vi "UI_Set_Play_State_(03A).vi"(3 "error in (no error)":errorcluster, 4 "Settings cluster in":T1={"Defaults"={"Default User"=0.0, "VISA Resource Name "=""}, "Recording and saving"={"Researcher name"="", "Name prefix"="", "Data filtering"=0, "Stop at"=0.0, "\"Stop at\" enabled"=FALSE}, "Geometry"={"Cage diameter, mm"=0, "Starting angle MIDFIELD"=0, "Starting angle BORDER"=0, "Radius, mm CENTER"=0, "Radius, mm MIDFIELD"=0, "N segments MIDFIELD"=0, "N segments BORDER"=0, "R-gap, mm"=0.0, "Bridge swap"=FALSE, "Bridge H. offset"=0.0, "Bridge V. offset"=0.0, "Twisted neck"=FALSE, "Alt. magn. orientation"=FALSE}, "IO parameters"={"IO general config."=0, "IO 1 configuration"=0, "IO 2 configuration"=0, "IO 3 configuration"=0, "IO 4 configuration"=0, "Activate ext. RS-232"=0, "IO inversion config."=0, "Sync capability"=1}, "Stimulus presets array"=[{"Event type"=0, "Dur., s"=0.0, "Stim., s"=0.0, "TTL out N"=1, "Set/Clear"=FALSE, "Stim. has been set"=FALSE}, {"Event type"=0, "Dur., s"=0.0, "Stim., s"=0.0, "TTL out N"=1, "Set/Clear"=FALSE, "Stim. has been set"=FALSE}, {"Event type"=0, "Dur., s"=0.0, "Stim., s"=0.0, "TTL out N"=1, "Set/Clear"=FALSE, "Stim. has been set"=FALSE}, {"Event type"=0, "Dur., s"=0.0, "Stim., s"=0.0, "TTL out N"=1, "Set/Clear"=FALSE, "Stim. has been set"=FALSE}, {"Event type"=0, "Dur., s"=0.0, "Stim., s"=0.0, "TTL out N"=1, "Set/Clear"=FALSE, "Stim. has been set"=FALSE}, {"Event type"=0, "Dur., s"=0.0, "Stim., s"=0.0, "TTL out N"=1, "Set/Clear"=FALSE, "Stim. has been set"=FALSE}, {"Event type"=0, "Dur., s"=0.0, "Stim., s"=0.0, "TTL out N"=1, "Set/Clear"=FALSE, "Stim. has been set"=FALSE}, {"Event type"=0, "Dur., s"=0.0, "Stim., s"=0.0, "TTL out N"=1, "Set/Clear"=FALSE, "Stim. has been set"=FALSE}, {"Event type"=0, "Dur., s"=0.0, "Stim., s"=0.0, "TTL out N"=1, "Set/Clear"=FALSE, "Stim. has been set"=FALSE}, {"Event type"=0, "Dur., s"=0.0, "Stim., s"=0.0, "TTL out N"=1, "Set/Clear"=FALSE, "Stim. has been set"=FALSE}, {"Event type"=0, "Dur., s"=0.0, "Stim., s"=0.0, "TTL out N"=1, "Set/Clear"=FALSE, "Stim. has been set"=FALSE}, {"Event type"=0, "Dur., s"=0.0, "Stim., s"=0.0, "TTL out N"=1, "Set/Clear"=FALSE, "Stim. has been set"=FALSE}, {"Event type"=0, "Dur., s"=0.0, "Stim., s"=0.0, "TTL out N"=1, "Set/Clear"=FALSE, "Stim. has been set"=FALSE}, {"Event type"=0, "Dur., s"=0.0, "Stim., s"=0.0, "TTL out N"=1, "Set/Clear"=FALSE, "Stim. has been set"=FALSE}], "Settings loaded OK"=FALSE} {"Stimulus presets array"."Event type" items=["Stay for N seconds"]; "Stimulus presets array"."TTL out N" items=["1"=1, "2"=2, "1+2"=3]; "Geometry"."Cage diameter, mm" scale=0.0..340.0}, 5 "All references in":T7) -> (0 "error out":errorcluster, 1 "Settings cluster out":T1={"Defaults"={"Default User"=0.0, "VISA Resource Name "=""}, "Recording and saving"={"Researcher name"="", "Name prefix"="", "Data filtering"=0, "Stop at"=0.0, "\"Stop at\" enabled"=FALSE}, "Geometry"={"Cage diameter, mm"=0, "Starting angle MIDFIELD"=0, "Starting angle BORDER"=0, "Radius, mm CENTER"=0, "Radius, mm MIDFIELD"=0, "N segments MIDFIELD"=0, "N segments BORDER"=0, "R-gap, mm"=0.0, "Bridge swap"=FALSE, "Bridge H. offset"=0.0, "Bridge V. offset"=0.0, "Twisted neck"=FALSE, "Alt. magn. orientation"=FALSE}, "IO parameters"={"IO general config."=0, "IO 1 configuration"=0, "IO 2 configuration"=0, "IO 3 configuration"=0, "IO 4 configuration"=0, "Activate ext. RS-232"=0, "IO inversion config."=0, "Sync capability"=1}, "Stimulus presets array"=[{"Event type"=0, "Dur., s"=0.0, "Stim., s"=0.0, "TTL out N"=1, "Set/Clear"=FALSE, "Stim. has been set"=FALSE}, {"Event type"=0, "Dur., s"=0.0, "Stim., s"=0.0, "TTL out N"=1, "Set/Clear"=FALSE, "Stim. has been set"=FALSE}, {"Event type"=0, "Dur., s"=0.0, "Stim., s"=0.0, "TTL out N"=1, "Set/Clear"=FALSE, "Stim. has been set"=FALSE}, {"Event type"=0, "Dur., s"=0.0, "Stim., s"=0.0, "TTL out N"=1, "Set/Clear"=FALSE, "Stim. has been set"=FALSE}, {"Event type"=0, "Dur., s"=0.0, "Stim., s"=0.0, "TTL out N"=1, "Set/Clear"=FALSE, "Stim. has been set"=FALSE}, {"Event type"=0, "Dur., s"=0.0, "Stim., s"=0.0, "TTL out N"=1, "Set/Clear"=FALSE, "Stim. has been set"=FALSE}, {"Event type"=0, "Dur., s"=0.0, "Stim., s"=0.0, "TTL out N"=1, "Set/Clear"=FALSE, "Stim. has been set"=FALSE}, {"Event type"=0, "Dur., s"=0.0, "Stim., s"=0.0, "TTL out N"=1, "Set/Clear"=FALSE, "Stim. has been set"=FALSE}, {"Event type"=0, "Dur., s"=0.0, "Stim., s"=0.0, "TTL out N"=1, "Set/Clear"=FALSE, "Stim. has been set"=FALSE}, {"Event type"=0, "Dur., s"=0.0, "Stim., s"=0.0, "TTL out N"=1, "Set/Clear"=FALSE, "Stim. has been set"=FALSE}, {"Event type"=0, "Dur., s"=0.0, "Stim., s"=0.0, "TTL out N"=1, "Set/Clear"=FALSE, "Stim. has been set"=FALSE}, {"Event type"=0, "Dur., s"=0.0, "Stim., s"=0.0, "TTL out N"=1, "Set/Clear"=FALSE, "Stim. has been set"=FALSE}, {"Event type"=0, "Dur., s"=0.0, "Stim., s"=0.0, "TTL out N"=1, "Set/Clear"=FALSE, "Stim. has been set"=FALSE}, {"Event type"=0, "Dur., s"=0.0, "Stim., s"=0.0, "TTL out N"=1, "Set/Clear"=FALSE, "Stim. has been set"=FALSE}], "Settings loaded OK"=FALSE} {"Stimulus presets array"."Event type" items=["Stay for N seconds"]; "Stimulus presets array"."TTL out N" items=["1"=1, "2"=2, "1+2"=3]; "Geometry"."Cage diameter, mm" scale=0.0..340.0}, 2 "All references out":T7)   [LabVIEW 2018]
uses:
  Controls/CTL_All_References.ctl
  Controls/CTL_Controls_References.ctl
  Controls/CTL_Indicators_References.ctl
  Controls/CTL_Panes_and_VIs_References.ctl
  Controls/CTL_Histogram_Properties.ctl
  <vilib>/Utility/miscctls.llb/LVRangeTypeDef.ctl
  Controls/CTL_Settings_cluster.ctl
  Controls/CTL_Segmented_plot_parameters.ctl
  Controls/CTL_IO_params_cluster.ctl
  Controls/CTL_Single_stimulus_setting.ctl
  <vilib>/Utility/error.llb/Error Cluster From Error Code.vi
  <vilib>/ErrorRing/Error Ring.xnode
panel:
  in  "Histogram initialization cluster":T5={"X Scale.Range"={"Minimum"=0.0, "Maximum"=13.0, "Increment"=1.0, "Minor Increment"=1.0, "Start"=0.0}, "Caption.Text"="Zone preference (normalized)", "X Scale.Offset and Multiplier:Multiplier"=1.0, "X Scale.Offset and Multiplier:Offset"=0.0, "X Scale.Scale Fit"=2, "X Scale.Display Format:Precision"=0, "Y Scale.Mapping Mode"=0, "Zones preference empty initialized array"=[0, 0, 0, 0, 0, 0, 0, 0, 0, 0, 0, 0, 0, 0], "Plot.Fill/Point Color"=15790320}
  out "Panes references":T10
  out "Controls references params":string[][](array[string])
  out "Indicators references params":string[][](array[string])
  out "Indicators references":T9
  out "Controls references":T8
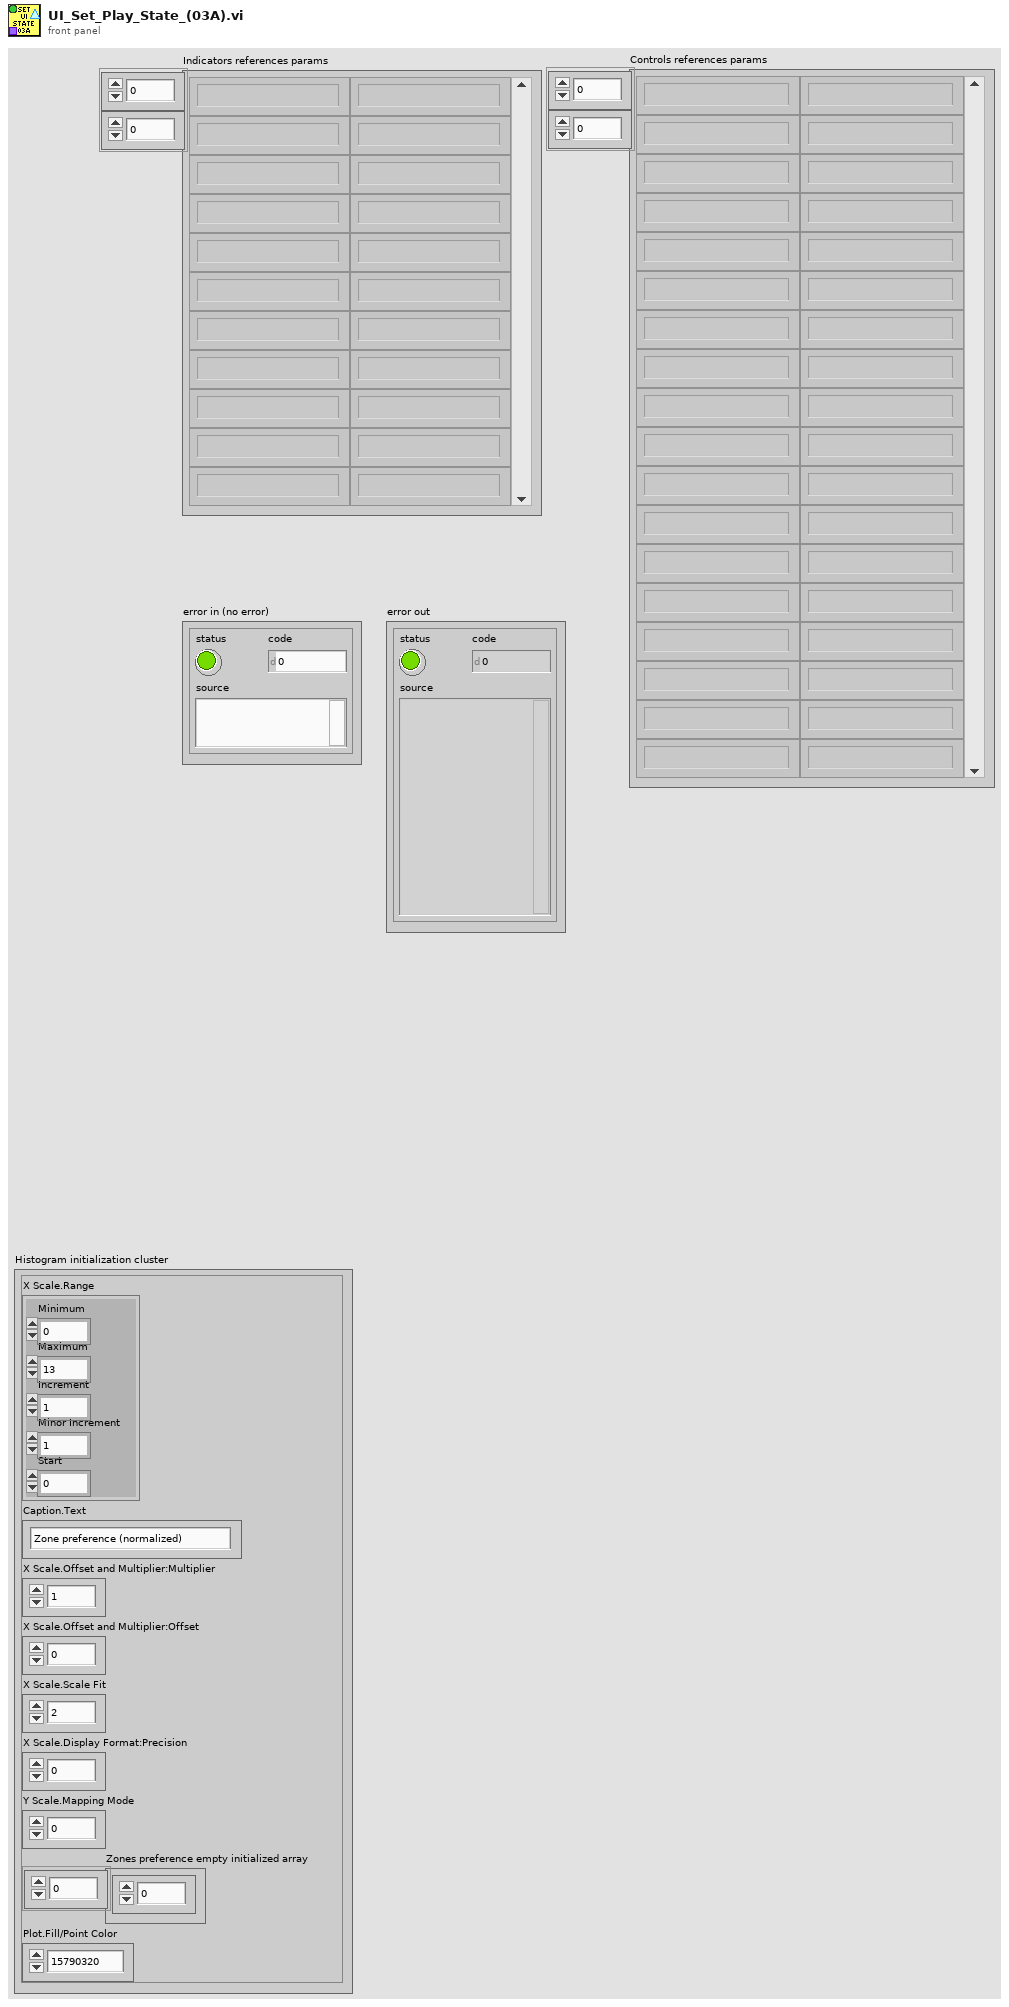
[diagram p1: front panel]
types:
  T1 = typedef "CTL_Settings_cluster.ctl" = cluster{"Defaults":cluster{"Default User":dbl, "VISA Resource Name ":string}, "Recording and saving":cluster{"Researcher name":string, "Name prefix":string, "Data filtering":u16, "Stop at":dbl, "\"Stop at\" enabled":bool}, "Geometry":T2, "IO parameters":T3, "Stimulus presets array":T4[], "Settings loaded OK":bool}
  T2 = typedef "CTL_Segmented_plot_parameters.ctl" = cluster{"Cage diameter, mm":u16, "Starting angle MIDFIELD":i16, "Starting angle BORDER":i16, "Radius, mm CENTER":u16, "Radius, mm MIDFIELD":u16, "N segments MIDFIELD":u8, "N segments BORDER":u8, "R-gap, mm":sgl, "Bridge swap":bool, "Bridge H. offset":sgl, "Bridge V. offset":sgl, "Twisted neck":bool, "Alt. magn. orientation":bool}
  T3 = typedef "CTL_IO_params_cluster.ctl" = cluster{"IO general config.":u16, "IO 1 configuration":u16, "IO 2 configuration":u16, "IO 3 configuration":u16, "IO 4 configuration":u16, "Activate ext. RS-232":u16, "IO inversion config.":u16, "Sync capability":u8}
  T4 = typedef "CTL_Single_stimulus_setting.ctl" = cluster{"Event type":u16, "Dur., s":sgl, "Stim., s":sgl, "TTL out N":u16, "Set/Clear":bool, "Stim. has been set":bool}
  T5 = typedef "CTL_Histogram_Properties.ctl" = cluster{"X Scale.Range":T6, "Caption.Text":string, "X Scale.Offset and Multiplier:Multiplier":dbl, "X Scale.Offset and Multiplier:Offset":dbl, "X Scale.Scale Fit":u8, "X Scale.Display Format:Precision":u8, "Y Scale.Mapping Mode":u8, "Zones preference empty initialized array":i32[], "Plot.Fill/Point Color":u32}
  T6 = typedef "LVRangeTypeDef.ctl" = cluster{"Minimum":dbl, "Maximum":dbl, "Increment":dbl, "Minor Increment":dbl, "Start":dbl}
  T7 = typedef "CTL_All_References.ctl" = cluster{"Controls references":T8, "Indicators references":T9, "Panes references":T10}
  T8 = typedef "CTL_Controls_References.ctl" = cluster{"Check HW connection":refnum<vi>, "Start Tracking button":refnum<vi>, "Reset zones":refnum<vi>, "Reset stimuli":refnum<vi>, "Record/Stop":refnum<vi>, "Reset barplot":refnum<vi>, "Multiplyer of chart RX":refnum<vi>, "Show zones":refnum<vi>, "Show magnets":refnum<vi>, "Show heatmap":refnum<vi>, "Show full track":refnum<vi>, "Open File":refnum<vi>, "Play/Pause":refnum<vi>, "Trace, s":refnum<vi>, "Playback speed":refnum<vi>, "Timeline":refnum<vi>, "By Zone stim. setup":refnum<vi>, "Set, Rec and Analyse Tab":refnum<vi>, "Cage radial segmentation":refnum<vi>, "Set IO config":refnum<vi>}
  T9 = typedef "CTL_Indicators_References.ctl" = cluster{"HW info":refnum<vi>, "Port":refnum<vi>, "Ready":refnum<vi>, "IO status indicator":refnum<vi>, "Current Time":refnum<vi>, "Record timestamp":refnum<vi>, "Mouse speed":refnum<vi>, "Mouse speed, mm/s":refnum<vi>, "Running, perc. of time":refnum<vi>, "Histograms":refnum<vi>, "Cage size":refnum<vi>}
  T10 = typedef "CTL_Panes_and_VIs_References.ctl" = cluster{"Pane":refnum<vi>, "This VI":refnum<vi>}
  T11 = enum8{"Enabled", "Disabled", "Disabled and Grayed Out"}
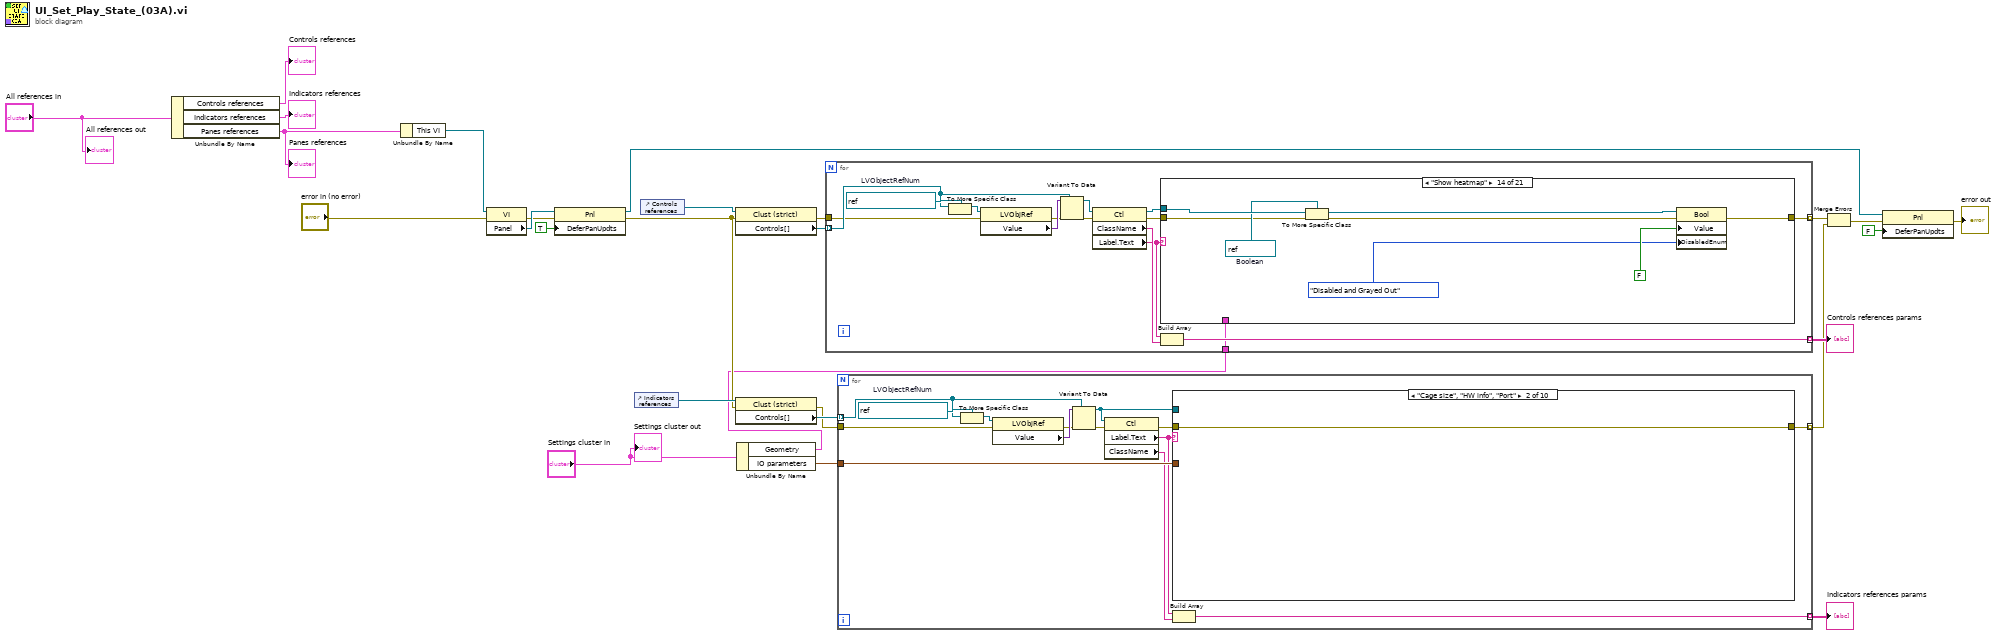
[diagram p0: block diagram]
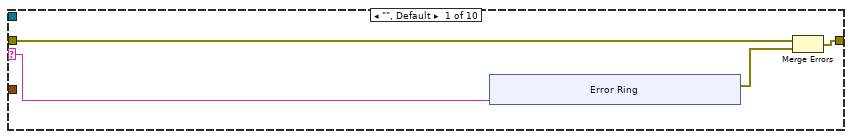
[diagram p2: hidden frame]
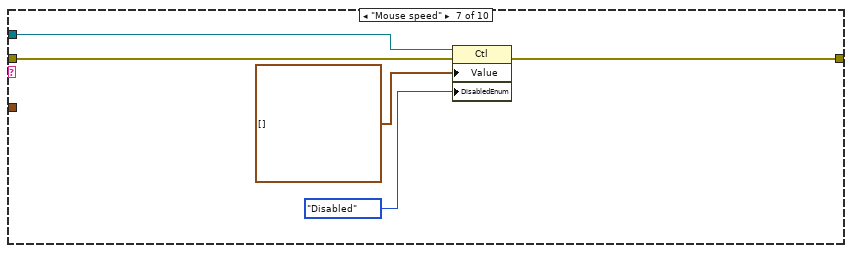
[diagram p7: hidden frame]
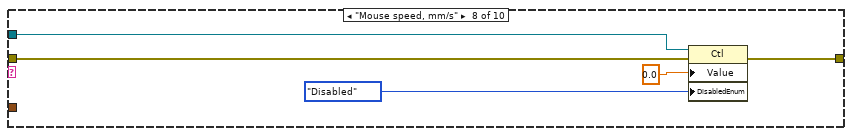
[diagram p8: hidden frame]
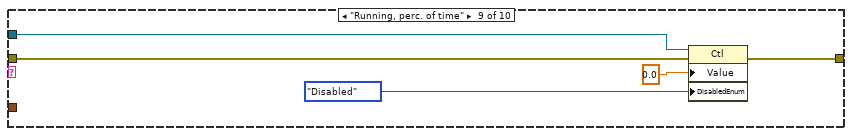
[diagram p9: hidden frame]
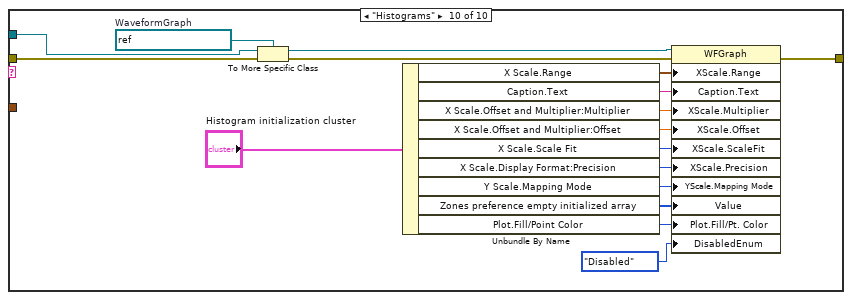
[diagram p10: hidden frame]
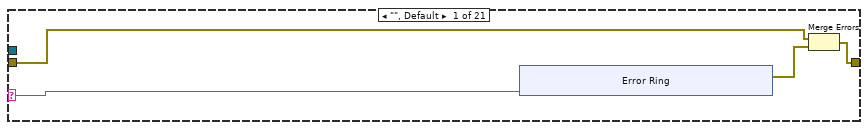
[diagram p11: hidden frame]
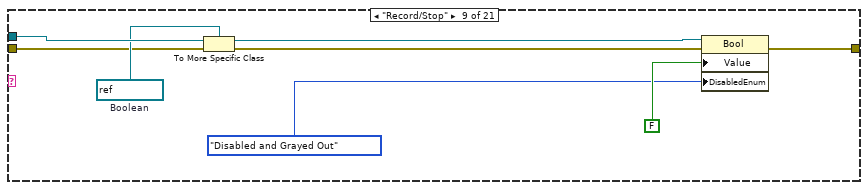
[diagram p19: hidden frame]
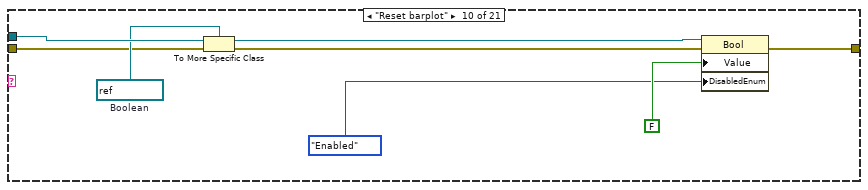
[diagram p20: hidden frame]
diagram:
  n1 = Unbundle By Name("All references in") -> ("Controls references"=→"Controls references":T8, "Indicators references"=→"Indicators references":T9, "Panes references"=w18:T10)
  "Panes references" <- w18
  n2 = Unbundle By Name(w18) -> ("This VI"=w15:refnum<vi>)
  n3 = property class="VI"(reference=w15, error in="error in (no error)") -> (error out=w7:errorcluster, "Panel"=w17:refnum<vi>)  [unwired: 1 out]
  n4 = property class="Pnl"(reference=w17, error in=w7, "DeferPanUpdts"=TRUE ("Defer Panel Updates")) -> (reference out=w8:refnum<vi>, error out=w14:errorcluster)
  n5 = control-ref of="Indicators references"() -> (w21:refnum<vi>)
  n6 = control-ref of="Controls references"() -> (w23:refnum<vi>)
  n7 = property class="Clust (strict)"(reference=w23, error in=w14) -> (error out=w13:errorcluster, "Controls[]"=w24:refnum<vi>[])  [unwired: 1 out]
  n8 = property class="Clust (strict)"(reference=w21, error in=w14) -> (error out=w12:errorcluster, "Controls[]"=w22:refnum<vi>[])  [unwired: 1 out]
  n9 = Unbundle By Name("Settings cluster in") -> ("Geometry"=w1:T2, "IO parameters"=w3:T3)
  n10 = for {
    tunnel: w24 -> [w39] mode=indexing
    tunnel: [w36] -> w19 mode=indexing
    tunnel: w13 -> [w35]
    tunnel: [w31] -> w5 mode=indexing
    tunnel: w1 -> [w28]
    w41 = refnum<vi> refnum  # LVObjectRefNum
    n11 = To More Specific Class(target class=w41, reference=w39) -> (specific class reference=w42:refnum<vi>)  [unwired: 1 in, 1 out]
    n12 = property class="LVObjRef"(reference=w42, error in=w35) -> (error out=w34:errorcluster, "Value"=w40:variant)  [unwired: 1 out]
    n13 = Variant To Data(error in=w34, type=w39, Variant=w40) -> (data=w38:refnum<vi>, error out=w33:errorcluster)
    n14 = property class="Ctl"(reference=w38, error in=w33) -> (reference out=w29:refnum<vi>, error out=w30:errorcluster, "ClassName"=w37:string, "Label.Text"=w32:string)
    n15 = case shown="\"Show heatmap\"" w32 {
      selector: w32 -> [w43 _ _ _ _ _ _ _ _ _ _ _ _ _ _ _ _ _ _ _ _]
      tunnel: [w45 w54 w55 w56 w57 w58 w59 w60 w63 w71 w79 w87 w93 w96 w104 w110 w111 w114 w122 w130 w136] -> w31
      tunnel: w30 -> [w46 w54 w55 w56 w57 w58 w59 w60 w65 w73 w81 w89 w93 w98 w106 w110 w111 w116 w124 w132 w136]
      tunnel: w29 -> [_ _ _ _ _ _ _ _ w68 w76 w84 w92 _ w101 w109 _ _ w119 w127 w135 _]
      tunnel: w28 -> [_ _ _ _ _ _ _ _ _ _ _ _ _ _ _ _ _ _ _ _ _]
      frame "", Default {
        n16 = xnode "Error Ring"("parameter 0"=w43) -> ("error out"=w44:errorcluster)
        n17 = Merge Errors(w46, w44) -> (w45:errorcluster)
      }
      frame "Cage radial segmentation" {
      }
      frame "Set/Rec and Analyse Tab" {
      }
      frame "Check HW connection" {
      }
      frame "Save settings" {
      }
      frame "Set IO config" {
      }
      frame "Reset zones" {
      }
      frame "Reset stimuli" {
      }
      frame "Record/Stop" {
        w67 = refnum<vi> refnum  # Boolean
        n18 = To More Specific Class(target class=w67, reference=w68, error in=w65) -> (specific class reference=w66:refnum<vi>, error out=w64:errorcluster)
        n19 = property class="Bool"(reference=w66, error in=w64, "Value"=FALSE, "DisabledEnum"=T11."Disabled and Grayed Out" ("Disabled")) -> (error out=w63:errorcluster)  [unwired: 1 out]
      }
      frame "Reset barplot" {
        w75 = refnum<vi> refnum  # Boolean
        n20 = To More Specific Class(target class=w75, reference=w76, error in=w73) -> (specific class reference=w74:refnum<vi>, error out=w72:errorcluster)
        n21 = property class="Bool"(reference=w74, error in=w72, "Value"=FALSE, "DisabledEnum"=T11."Enabled" ("Disabled")) -> (error out=w71:errorcluster)  [unwired: 1 out]
      }
      frame "Multiplyer of chart RX" {
        w83 = refnum<vi> refnum  # Slide
        n22 = To More Specific Class(target class=w83, reference=w84, error in=w81) -> (specific class reference=w82:refnum<vi>, error out=w80:errorcluster)
        n23 = property class="Slide"(reference=w82, error in=w80, "Value"=u8 1, "DisabledEnum"=T11."Enabled" ("Disabled")) -> (error out=w79:errorcluster)  [unwired: 1 out]
      }
      frame "Show zones" {
        w91 = refnum<vi> refnum  # Boolean
        n24 = To More Specific Class(target class=w91, reference=w92, error in=w89) -> (specific class reference=w90:refnum<vi>, error out=w88:errorcluster)
        n25 = property class="Bool"(reference=w90, error in=w88, "Value"=TRUE, "DisabledEnum"=T11."Enabled" ("Disabled")) -> (error out=w87:errorcluster)  [unwired: 1 out]
      }
      frame "Show magnets" {
      }
      frame "Show heatmap" {
        w100 = refnum<vi> refnum  # Boolean
        n26 = To More Specific Class(target class=w100, reference=w101, error in=w98) -> (specific class reference=w99:refnum<vi>, error out=w97:errorcluster)
        n27 = property class="Bool"(reference=w99, error in=w97, "Value"=FALSE, "DisabledEnum"=T11."Disabled and Grayed Out" ("Disabled")) -> (error out=w96:errorcluster)  [unwired: 1 out]
      }
      frame "Show full track" {
        w108 = refnum<vi> refnum  # Boolean
        n28 = To More Specific Class(target class=w108, reference=w109, error in=w106) -> (specific class reference=w107:refnum<vi>, error out=w105:errorcluster)
        n29 = property class="Bool"(reference=w107, error in=w105, "Value"=FALSE, "DisabledEnum"=T11."Disabled and Grayed Out" ("Disabled")) -> (error out=w104:errorcluster)  [unwired: 1 out]
      }
      frame "Open File" {
      }
      frame "Play/Pause" {
      }
      frame "Trace, s" {
        w118 = refnum<vi> refnum  # Slide
        n30 = To More Specific Class(target class=w118, reference=w119, error in=w116) -> (specific class reference=w117:refnum<vi>, error out=w115:errorcluster)
        n31 = property class="Slide"(reference=w117, error in=w115, "Value"=u8 5, "DisabledEnum"=T11."Enabled" ("Disabled")) -> (error out=w114:errorcluster)  [unwired: 1 out]
      }
      frame "Playback speed" {
        w126 = refnum<vi> refnum  # Ring
        n32 = To More Specific Class(target class=w126, reference=w127, error in=w124) -> (specific class reference=w125:refnum<vi>, error out=w123:errorcluster)
        n33 = property class="Ring"(reference=w125, error in=w123, "Value"=u8 3, "DisabledEnum"=T11."Disabled and Grayed Out" ("Disabled")) -> (error out=w122:errorcluster)  [unwired: 1 out]
      }
      frame "Timeline" {
        w134 = refnum<vi> refnum  # Slide
        n34 = To More Specific Class(target class=w134, reference=w135, error in=w132) -> (specific class reference=w133:refnum<vi>, error out=w131:errorcluster)
        n35 = property class="Slide"(reference=w133, error in=w131, "Value"=u8 5, "DisabledEnum"=T11."Disabled" ("Disabled")) -> (error out=w130:errorcluster)  [unwired: 1 out]
      }
      frame "By Zone stim. setup" {
      }
    }
    n36 = Build Array(w32, w37) -> (w36:string[])
  }
  "Controls references params" <- w19
  n37 = for {
    tunnel: w22 -> [w147] mode=indexing
    tunnel: [w137] -> w20 mode=indexing
    tunnel: w12 -> [w145]
    tunnel: [w141] -> w11 mode=indexing
    tunnel: w3 -> [w140]
    w149 = refnum<vi> refnum  # LVObjectRefNum
    n38 = To More Specific Class(target class=w149, reference=w147) -> (specific class reference=w150:refnum<vi>)  [unwired: 1 in, 1 out]
    n39 = property class="LVObjRef"(reference=w150, error in=w145) -> (error out=w144:errorcluster, "Value"=w148:variant)  [unwired: 1 out]
    n40 = Variant To Data(error in=w144, type=w147, Variant=w148) -> (data=w146:refnum<vi>, error out=w143:errorcluster)
    n41 = property class="Ctl"(reference=w146, error in=w143) -> (error out=w142:errorcluster, "Label.Text"=w139:string, "ClassName"=w138:string)  [unwired: 1 out]
    n42 = case shown="\"Cage size\", \"HW info\", \"Port\"" w139 {
      selector: w139 -> [w151 _ _ _ _ _ _ _ _ _]
      tunnel: w146 -> [_ _ _ _ _ _ w171 w176 w181 w198]
      tunnel: w142 -> [w154 w162 w163 w164 w165 w166 w170 w175 w180 w184]
      tunnel: [w153 w162 w163 w164 w165 w166 w169 w174 w179 w197] -> w141
      tunnel: w140 -> [_ _ _ _ _ _ _ _ _ _]
      frame "", Default {
        n43 = xnode "Error Ring"("parameter 0"=w151) -> ("error out"=w152:errorcluster)
        n44 = Merge Errors(w154, w152) -> (w153:errorcluster)
      }
      frame "Cage size", "HW info", "Port" {
      }
      frame "Ready" {
      }
      frame "IO status indicator" {
      }
      frame "Current Time" {
      }
      frame "Record timestamp" {
      }
      frame "Mouse speed" {
        n45 = property class="Ctl"(reference=w171, error in=w170, "Value"=waveform(dbl)[] [] ("History Data"), "DisabledEnum"=T11."Disabled" ("Disabled")) -> (error out=w169:errorcluster)  [unwired: 1 out]
      }
      frame "Mouse speed, mm/s" {
        n46 = property class="Ctl"(reference=w176, error in=w175, "Value"=0.0, "DisabledEnum"=T11."Disabled" ("Disabled")) -> (error out=w174:errorcluster)  [unwired: 1 out]
      }
      frame "Running, perc. of time" {
        n47 = property class="Ctl"(reference=w181, error in=w180, "Value"=0.0, "DisabledEnum"=T11."Disabled" ("Disabled")) -> (error out=w179:errorcluster)  [unwired: 1 out]
      }
      frame "Histograms" {
        w195 = refnum<vi> refnum  # WaveformGraph
        n48 = To More Specific Class(target class=w195, reference=w198, error in=w184) -> (specific class reference=w196:refnum<vi>, error out=w183:errorcluster)
        n49 = Unbundle By Name("Histogram initialization cluster") -> ("X Scale.Range"=w193:T6, "Caption.Text"=w192:string, "X Scale.Offset and Multiplier:Multiplier"=w191:dbl, "X Scale.Offset and Multiplier:Offset"=w190:dbl, "X Scale.Scale Fit"=w189:u8, "X Scale.Display Format:Precision"=w188:u8, "Y Scale.Mapping Mode"=w187:u8, "Zones preference empty initialized array"=w186:i32[], "Plot.Fill/Point Color"=w185:u32)
        n50 = property class="WFGraph"(reference=w196, error in=w183, "XScale.Range"=w193, "Caption.Text"=w192, "XScale.Multiplier"=w191, "XScale.Offset"=w190, "XScale.ScaleFit"=w189, "XScale.Precision"=w188, "YScale.Mapping Mode"=w187, "Value"=w186, "Plot.Fill/Pt. Color"=w185, "DisabledEnum"=T11."Disabled" ("Disabled")) -> (error out=w197:errorcluster)  [unwired: 1 out]
      }
    }
    n51 = Build Array(w139, w138) -> (w137:string[])
  }
  "Indicators references params" <- w20
  n52 = Merge Errors(w5, w11) -> (w10:errorcluster)
  n53 = property class="Pnl"(reference=w8, error in=w10, "DeferPanUpdts"=FALSE ("Defer Panel Updates")) -> (error out=→"error out":errorcluster)  [unwired: 1 out]
  "All references out" <- "All references in"
  "Settings cluster out" <- "Settings cluster in"
